vi "B2G1_sqlite_createtable.vi"(8 "error in (no error)":errorcluster, 11 "Database File":string) -> (0 "error out":errorcluster)   [LabVIEW 2011]
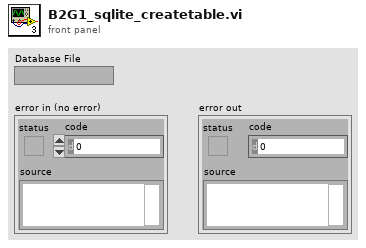
[diagram p1: front panel]
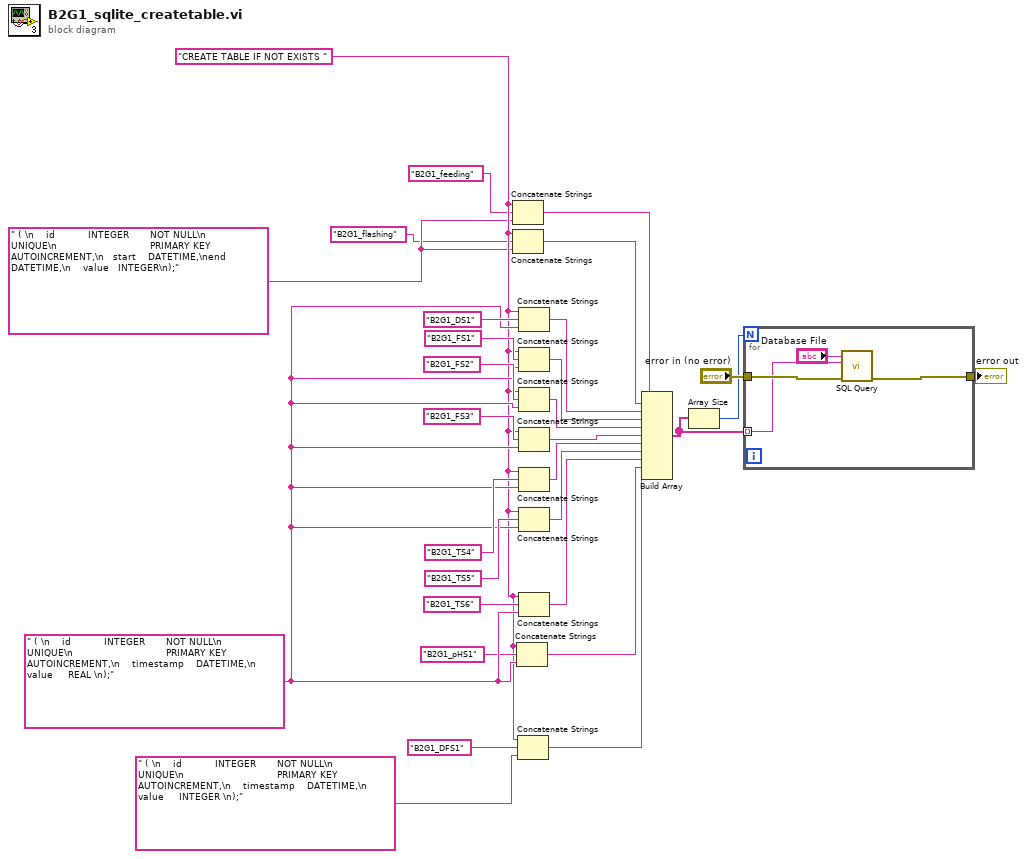
[diagram p0: block diagram]
diagram:
  w8 = " ( \n    id           INTEGER       NOT NULL\n                               UNIQUE\n                               PRIMARY KEY AUTOINCREMENT,\n    timestamp    DATETIME,\n    value     REAL \n);" ("SQL Query")
  w4 = "CREATE TABLE IF NOT EXISTS " ("SQL Query")
  w3 = " ( \n    id           INTEGER       NOT NULL\n                               UNIQUE\n                               PRIMARY KEY AUTOINCREMENT,\n   start    DATETIME,\nend    DATETIME,\n    value   INTEGER\n);" ("SQL Query")
  n1 = Concatenate Strings(w4, "B2G1_feeding" ("SQL Query"), w3) -> (w5:string)
  n2 = Concatenate Strings(w4, "B2G1_flashing" ("SQL Query"), w3) -> (w6:string)
  n3 = Concatenate Strings(w4, "B2G1_pHS1" ("SQL Query"), w8) -> (w9:string)
  n4 = Concatenate Strings(w4, "B2G1_DFS1" ("SQL Query"), " ( \n    id           INTEGER       NOT NULL\n                               UNIQUE\n                               PRIMARY KEY AUTOINCREMENT,\n    timestamp    DATETIME,\n    value     INTEGER \n);" ("SQL Query")) -> (w11:string)
  n5 = Concatenate Strings(w4, "B2G1_DS1" ("SQL Query"), w8) -> (w26:string)
  n6 = Concatenate Strings(w4, "B2G1_FS1" ("SQL Query"), w8) -> (w24:string)
  n7 = Concatenate Strings(w4, "B2G1_FS2" ("SQL Query"), w8) -> (w21:string)
  n8 = Concatenate Strings(w4, "B2G1_FS3" ("SQL Query"), w8) -> (w20:string)
  n9 = Concatenate Strings(w4, "B2G1_TS4" ("SQL Query"), w8) -> (w17:string)
  n10 = Concatenate Strings(w4, "B2G1_TS5" ("SQL Query"), w8) -> (w16:string)
  n11 = Concatenate Strings(w4, "B2G1_TS6" ("SQL Query"), w8) -> (w15:string)
  n12 = Build Array(w5, w6, w26, w24, w21, w20, w17, w16, w15, w9, w11) -> (w28:string[])
  n13 = Array Size(array=w28) -> (size(s)=w29:i32)
  n14 = for {
    N: w29 -> [_]
    tunnel: "error in (no error)" -> [w34]
    tunnel: w28 -> [w33] mode=indexing
    tunnel: [w32] -> w27
    n15 = call "SQL Query.vi"("error in (no error)"=w34, "SQL Query"=w33, "Database File"="Database File") -> ("error out"=w32:errorcluster)  [unwired: 6 in, 2 out]
  }
  "error out" <- w27
